vi "RT_SPI Host.vi"() -> ()   [LabVIEW 2019]
uses:
  <vilib>/FPGAPlugInAG/myRIO-1900/niLvFpga_Open_myRIO-1900.vi
  <vilib>/rvi/interface/common/dynamic/niFpgaDynamicAddResources.vi
  <vilib>/FPGAPlugInAG/Dynamic/niLvFpga_Close_Dynamic.vi
  <vilib>/rvi/interface/nirviOpenFPGA/nirviOpenFPGA.xnode
  FPGA Bitfiles/gpass2_FPGATarget_SPIFPGA_D2NdEaqdS6g.lvbitx
  SPI FPGA.vi
  <vilib>/rvi/interface/nirviCloseFPGA/nirviCloseFPGA.xnode
  <vilib>/IEDriver/SPIandI2C/Host/SPI/SPI Host.lvlib
panel:
  out "Readings to degree":dbl
  out "Waveform Chart":dbl(graph)
  out "Decimal Position":u16
  out "14 bit":u16 format="%b"
  out "16 bit":u16 format="%b"
  in  "stop":bool
  in  "Write Data":u8[](array[numeric])=[0, 0, 0, 0, 0, 0] format="%.0x"
  out "Read Data":u8[](array[numeric])=[115, 70] format="%b"
  in  "CS Active State":bool
  in  "Timeout (10 s)":u8=10
  in  "FPGA Clock (40 MHz)":u32=2000000
  in  "Port Number":u8
  in  "Number of Bits":u16=16
  in  "Chip Select":T1(ring)
  in  "Clock Rate":u32=100
  in  "Mode":u8
  # "Configuration"
  # "Write & Read"
  # "This example demonstrates how to use SPI driver to communicate with SPI device.\nThis example is intentionally broken until you compile this example for a specific target."
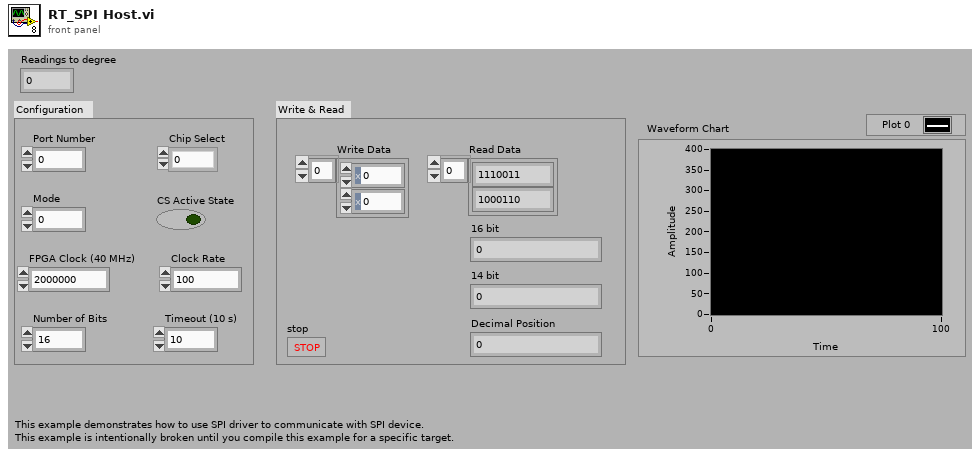
[diagram p1: front panel]
types:
  T1 = enum16{"0", "1", "2", "3", "4", "5", "6", "7", "8", "9"}
  T2 = cluster{"FPGA VI Reference":refnum<k20>, "Port Number":u8}
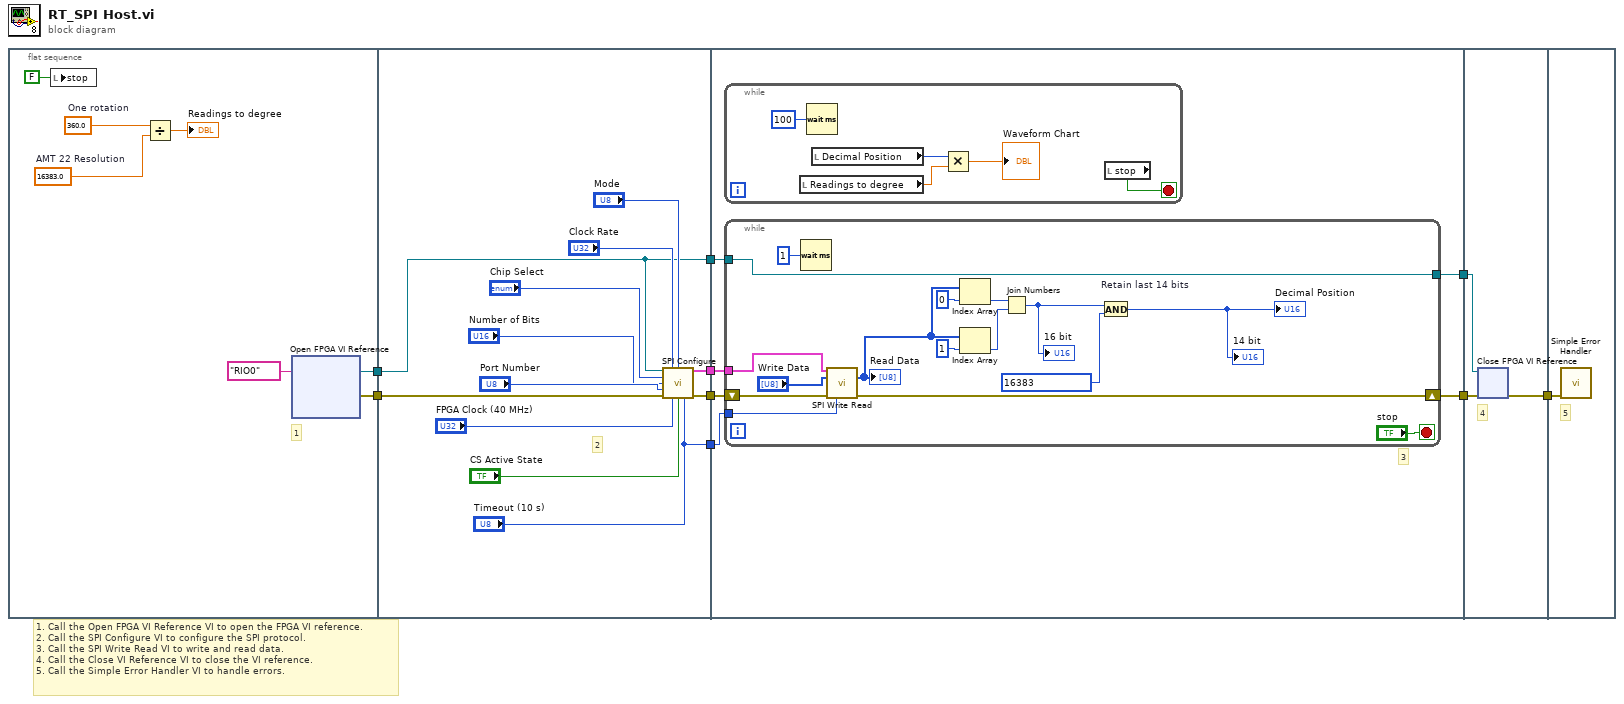
[diagram p0: block diagram]
diagram:
  # "1. Call the Open FPGA VI Reference VI to open the FPGA VI reference.\n2. Call the SPI Configure VI to configure the SPI protocol.\n3. Call the SPI Write Read VI to write and read data.\n4. Call the Close VI Reference VI to close the VI reference.\n5. Call the Simple Error Handler VI to handle errors."
  n1 = flat-sequence {
    tunnel: [w16] -> w6
    tunnel: [w15] -> w5
    tunnel: [w18] -> w9
    tunnel: [w19] -> w8
    tunnel: ["Timeout (10 s)"] -> w7
    tunnel: w6 -> [w21]
    tunnel: w5 -> [w17]
    tunnel: [w17] -> w4
    tunnel: w9 -> [w34]
    tunnel: w8 -> [w33]
    tunnel: w7 -> [w31]
    tunnel: w4 -> [w29]
    tunnel: [w32] -> w3
    tunnel: [w30] -> w2
    tunnel: w3 -> [w58]
    tunnel: w2 -> [w56]
    tunnel: [w57] -> w1
    tunnel: w1 -> [w59]
    frame #0 {
      w11 = 16383.0  # AMT 22 Resolution
      w12 = 360.0  # One rotation
      # "1"
      n2 = local write "stop"(FALSE ("stop")) -> ()
      n3 = Divide(x=w12, y=w11) -> (x/y=→"Readings to degree":dbl)
      n4 = xnode "Open FPGA VI Reference"("resource name"=tag "RIO0") -> ("FPGA VI Reference Out"=w15:refnum<k20>, "error out"=w16:errorcluster)  [unwired: 1 in]
    }
    frame #1 {
      # "2"
      n5 = call <vilib>:"SPI Configure.vi"("FPGA VI Reference"=w17, "Clock Rate"="Clock Rate", "Mode"="Mode", "Chip Select"="Chip Select", "Number of Bits"="Number of Bits", "Port Number"="Port Number", "error in (no error)"=w21, "FPGA Clock (40 MHz)"="FPGA Clock (40 MHz)", "CS Active State"="CS Active State", "Timeout (10 s)"="Timeout (10 s)") -> ("FPGA Information Out"=w19:T2, "error out"=w18:errorcluster)  [unwired: 4 in]
    }
    frame #2 {
      # "3"
      n6 = while {
        stop <- w39 stop-if-true
        n7 = local read "Readings to degree"() -> (w36:dbl)
        n8 = Wait (ms)(milliseconds to wait=u32 100) -> ()  [unwired: 1 out]
        n9 = local read "Decimal Position"() -> (w37:u16)
        n10 = Multiply(x=w37, y=w36) -> (x*y=→"Waveform Chart":dbl)
        n11 = local read "stop"() -> (w39:bool)
      }
      n12 = while {
        tunnel: w33 -> [w49]
        tunnel: w31 -> [w47]
        shift-right: [w46] -> w32
        shift-left: w34 -> [w48]
        tunnel: [w55] -> w30
        tunnel: w29 -> [w55]
        stop <- "stop" stop-if-true
        n13 = Wait (ms)(milliseconds to wait=u32 1) -> ()  [unwired: 1 out]
        n14 = call <vilib>:"SPI Write Read.vi"("FPGA Information In"=w49, "Write Data"="Write Data", "error in (no error)"=w48, "Timeout (10 s)"=w47) -> ("Read Data"=w44:u8[], "error out"=w46:errorcluster)  [unwired: 9 in, 1 out]
        "Read Data" <- w44
        n15 = Index Array(array=w44, index=0) -> (element=w51:u8)
        n16 = Index Array(array=w44, index=1) -> (element=w50:u8)
        n17 = Join Numbers(hi=w51, lo=w50) -> ((hi.lo)=w42:u16)
        "16 bit" <- w42
        n18 = And "Retain last 14 bits"(x=w42, y=u16 16383) -> (x .and. y?=→"14 bit" →"Decimal Position":u16)
      }
    }
    frame #3 {
      # "4"
      n19 = xnode "Close FPGA VI Reference"("FPGA VI Reference In"=w56, "error in"=w58) -> ("error out"=w57:errorcluster)
    }
    frame #4 {
      # "5"
      n20 = call <vilib>:"Simple Error Handler.vi"("error in (no error)"=w59) -> ()  [unwired: 4 in, 5 out]
    }
  }
